vi "chooseCubeFloor.vi"(10 "cnt":i32, 11 "Type":enum16{"Z", "I", "O", "S", "L", "J", "T", "N"}(ring)) -> (3 "d":enum16{"Cube", "Floor"}(ring))   [LabVIEW 2018]
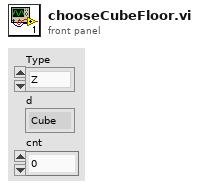
[diagram p1: front panel]
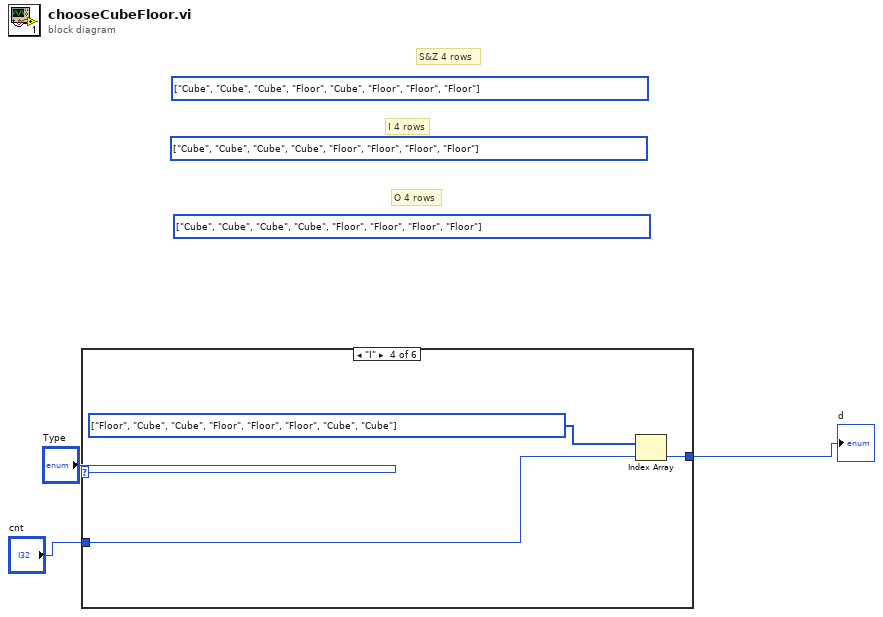
[diagram p0: block diagram]
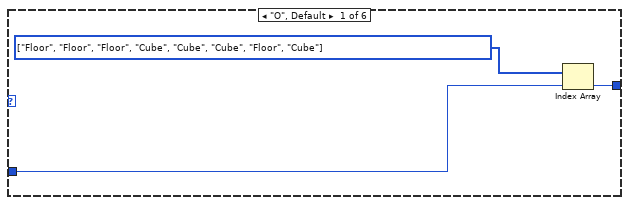
[diagram p2: hidden frame]
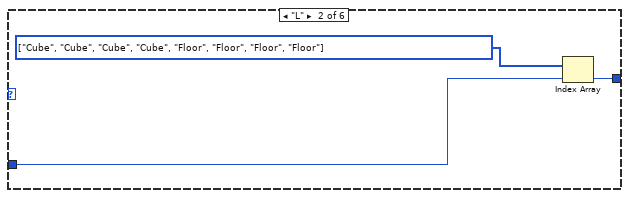
[diagram p3: hidden frame]
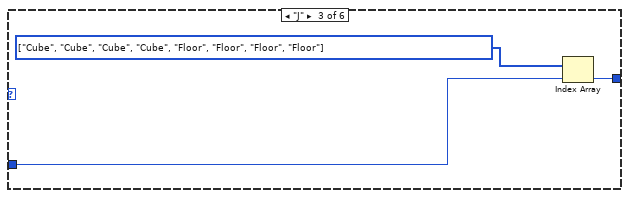
[diagram p4: hidden frame]
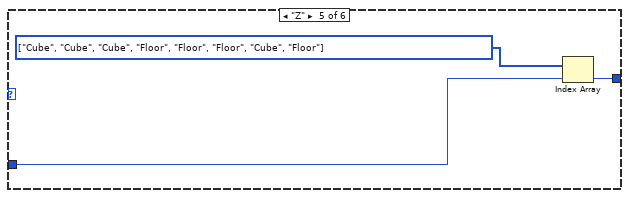
[diagram p5: hidden frame]
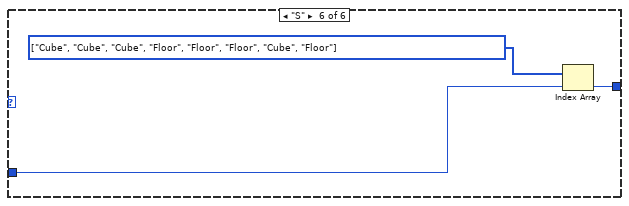
[diagram p6: hidden frame]
diagram:
  (unwired) enum16{"Cube", "Floor"}[] [enum."Cube", enum."Cube", enum."Cube", enum."Floor", enum."Cube", enum."Floor", enum."Floor", enum."Floor"] items=["Cube", "Floor"] ("d")
  (unwired) enum16{"Cube", "Floor"}[] [enum."Cube", enum."Cube", enum."Cube", enum."Cube", enum."Floor", enum."Floor", enum."Floor", enum."Floor"] items=["Cube", "Floor"] ("d")
  (unwired) enum16{"Cube", "Floor"}[] [enum."Cube", enum."Cube", enum."Cube", enum."Cube", enum."Floor", enum."Floor", enum."Floor", enum."Floor"] items=["Cube", "Floor"] ("d")
  # "S&Z 4 rows"
  # "I 4 rows"
  # "O 4 rows"
  n1 = case shown="\"I\"" "Type" {
    tunnel: "cnt" -> [w6 w9 w12 w15 w18 w21]
    tunnel: [w5 w8 w11 w14 w17 w20] -> w1
    frame "O", Default {
      w4 = enum16{"Cube", "Floor"}[] [enum."Floor", enum."Floor", enum."Floor", enum."Cube", enum."Cube", enum."Cube", enum."Floor", enum."Cube"] items=["Cube", "Floor"] ("d")
      n2 = Index Array(array=w4, index=w6) -> (element=w5:enum16{"Cube", "Floor"})
    }
    frame "L" {
      w7 = enum16{"Cube", "Floor"}[] [enum."Cube", enum."Cube", enum."Cube", enum."Cube", enum."Floor", enum."Floor", enum."Floor", enum."Floor"] items=["Cube", "Floor"] ("d")
      n3 = Index Array(array=w7, index=w9) -> (element=w8:enum16{"Cube", "Floor"})
    }
    frame "J" {
      w10 = enum16{"Cube", "Floor"}[] [enum."Cube", enum."Cube", enum."Cube", enum."Cube", enum."Floor", enum."Floor", enum."Floor", enum."Floor"] items=["Cube", "Floor"] ("d")
      n4 = Index Array(array=w10, index=w12) -> (element=w11:enum16{"Cube", "Floor"})
    }
    frame "I" {
      w13 = enum16{"Cube", "Floor"}[] [enum."Floor", enum."Cube", enum."Cube", enum."Floor", enum."Floor", enum."Floor", enum."Cube", enum."Cube"] items=["Cube", "Floor"] ("d")
      n5 = Index Array(array=w13, index=w15) -> (element=w14:enum16{"Cube", "Floor"})
    }
    frame "Z" {
      w16 = enum16{"Cube", "Floor"}[] [enum."Cube", enum."Cube", enum."Cube", enum."Floor", enum."Floor", enum."Floor", enum."Cube", enum."Floor"] items=["Cube", "Floor"] ("d")
      n6 = Index Array(array=w16, index=w18) -> (element=w17:enum16{"Cube", "Floor"})
    }
    frame "S" {
      w19 = enum16{"Cube", "Floor"}[] [enum."Cube", enum."Cube", enum."Cube", enum."Floor", enum."Floor", enum."Floor", enum."Cube", enum."Floor"] items=["Cube", "Floor"] ("d")
      n7 = Index Array(array=w19, index=w21) -> (element=w20:enum16{"Cube", "Floor"})
    }
  }
  "d" <- w1
